vi "InputToArray.vi"(8 "error in (no error)":errorcluster, 9 "Position":dbl, 10 "Axis":string) -> (0 "error out":errorcluster, 1 "Position Array":dbl[](array[numeric]), 2 "Axis Array":string[](array[string]))   [LabVIEW 2020]
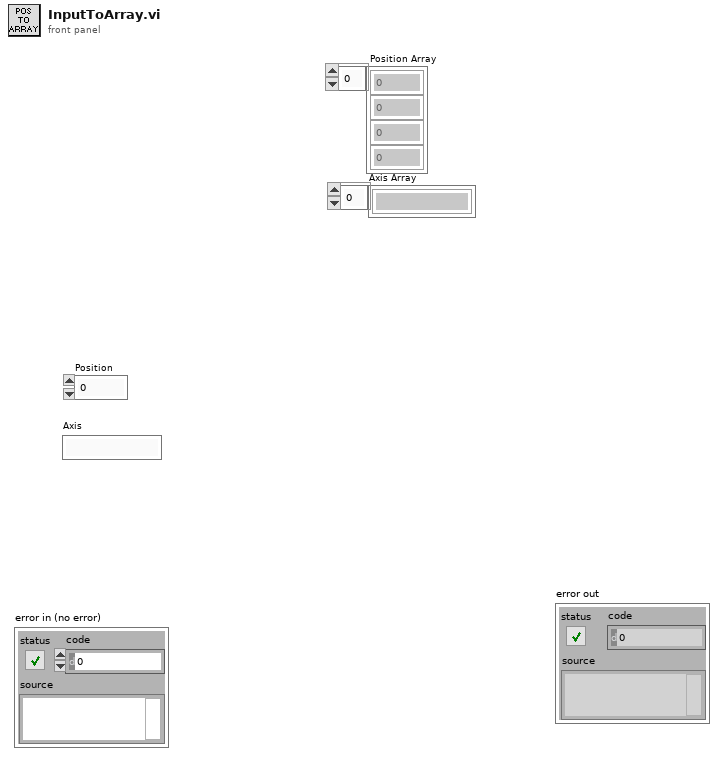
[diagram p1: front panel]
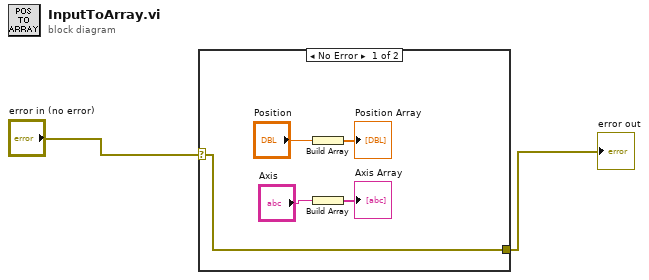
[diagram p0: block diagram]
diagram:
  n1 = case shown="No Error" "error in (no error)" {
    selector: "error in (no error)" -> [w3 w8]
    tunnel: [w3 w8] -> w1
    frame No Error {
      n2 = Build Array("Position") -> (→"Position Array":dbl[])
      n3 = Build Array("Axis") -> (→"Axis Array":string[])
    }
    frame Error {
    }
  }
  "error out" <- w1
